vi "Read loop condition.vi"(9 "Loop in":refnum<class "Loop.lvclass">) -> (3 "Loop out":refnum<class "Loop.lvclass">, 4 "conditional terminal":refnum<class "Terminal.lvclass">)   [LabVIEW 2014, in "Raspberry Pi Compatible Compiler for LabVIEW.lvlib" / "Loop.lvclass"]
uses:
  Loop.lvclass
  Terminal/Terminal.lvclass
  Loop.lvclass/Loop.ctl
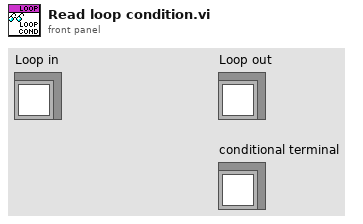
[diagram p1: front panel]
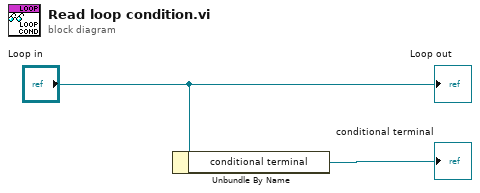
[diagram p0: block diagram]
diagram:
  n1 = Unbundle By Name("Loop in") -> ("conditional terminal"=→"conditional terminal":refnum<class "Terminal.lvclass">)
  "Loop out" <- "Loop in"
